vi "PCO Edge_Settings.vi"(10 "Buffers":i16[](array[numeric]), 11 "Handle":u64) -> (3 "Handle Out":u64)   [LabVIEW 2015]
panel:
  in  "Pixel correction":bool
  in  "OK Button":bool
  in  "Pixel clock":u32(ring)=286000000 items=["286MHz"=286000000, "95MHz"=95000000]
  in  "Shutter":u32(ring)=1 items=["Global"=2, "Rolling"=1]
  in  "Binning":u16[](array[numeric])
  in  "ROI":u16[][](array[numeric])
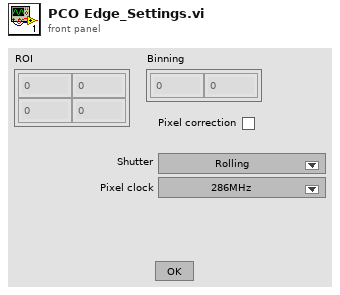
[diagram p1: front panel]
types:
  T1 = cluster{"SSize":u16, "CamType":u16, "CamsSubType":u16, "SerialNumber":u32, "HWVersion":u32, "FWVersion ":u32, "InterfaceType":u16, "HardwareVersions":cluster{"Board":u16, cluster{"string":string, "BatchNumber":u16, "MinorRevision":u8, "MajorRevision":u8, "Variant":u16}[]}, "FirmwareVersions":cluster{"DeviceNum":u16, cluster{"string":string, "MinorRevision":u8, "MajorRevision":u8, "Variant":u16}[]}}
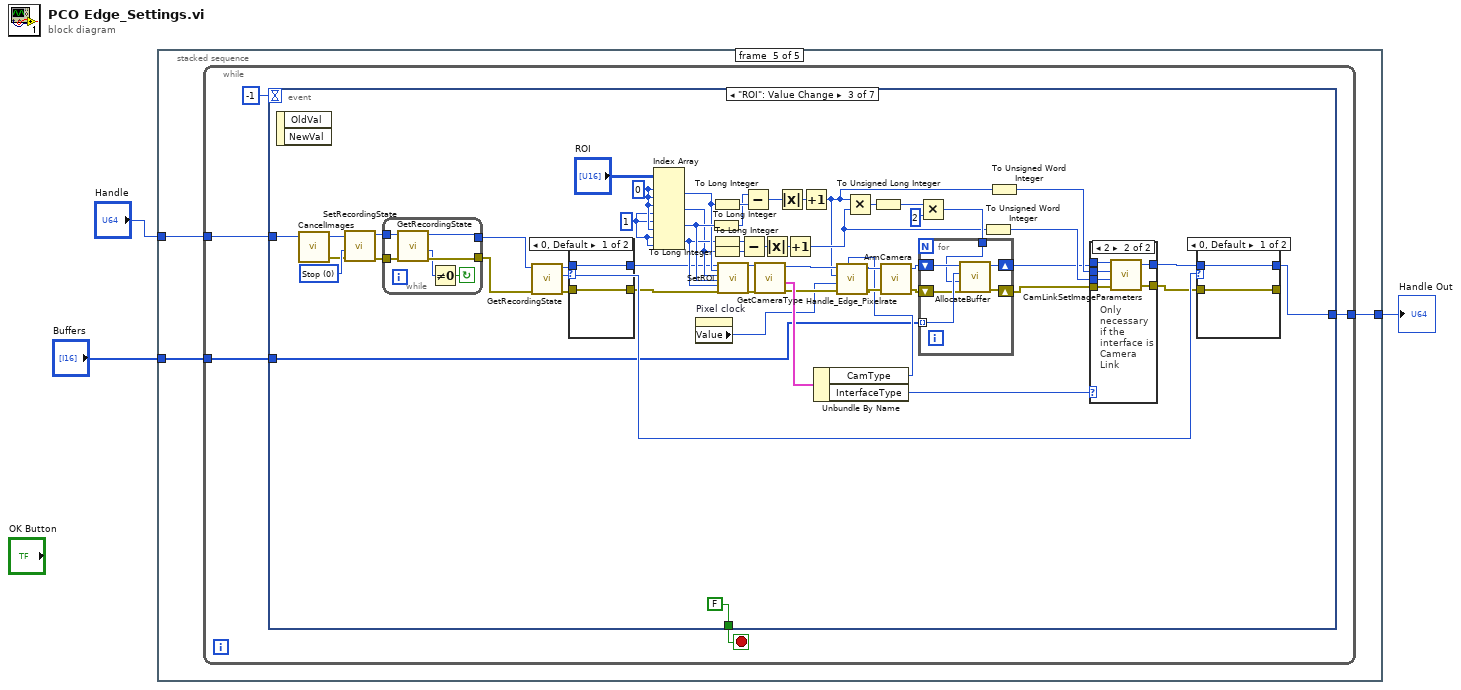
[diagram p0: block diagram]
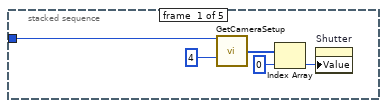
[diagram p2: hidden frame]
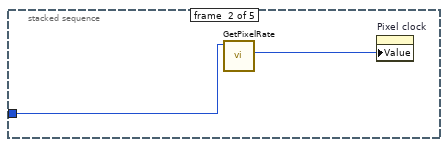
[diagram p3: hidden frame]
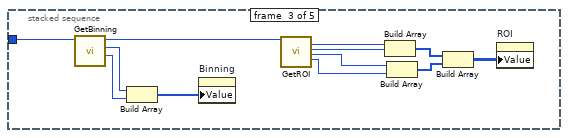
[diagram p4: hidden frame]
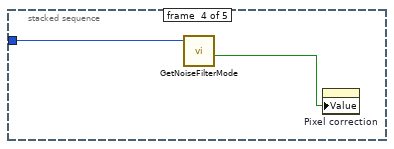
[diagram p5: hidden frame]
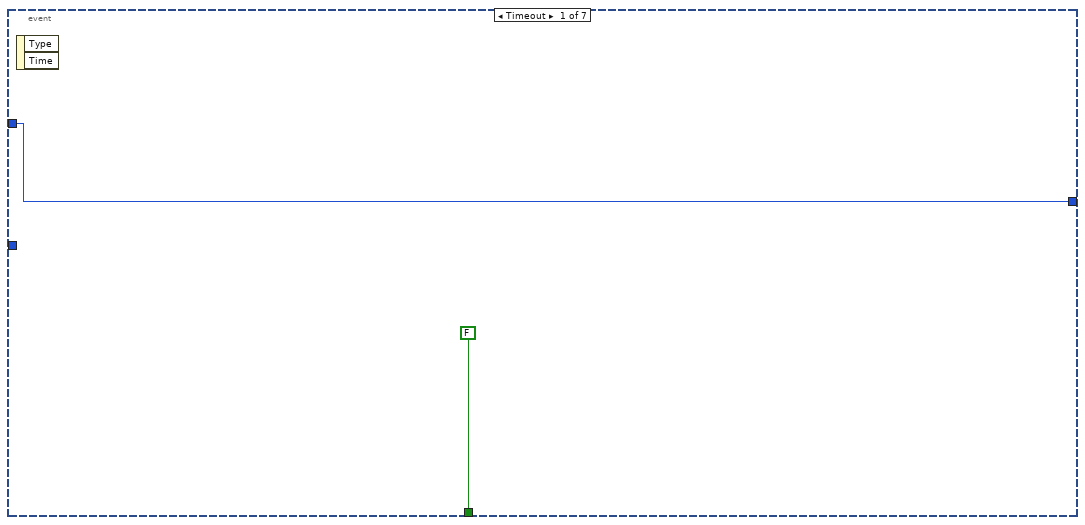
[diagram p6: hidden frame]
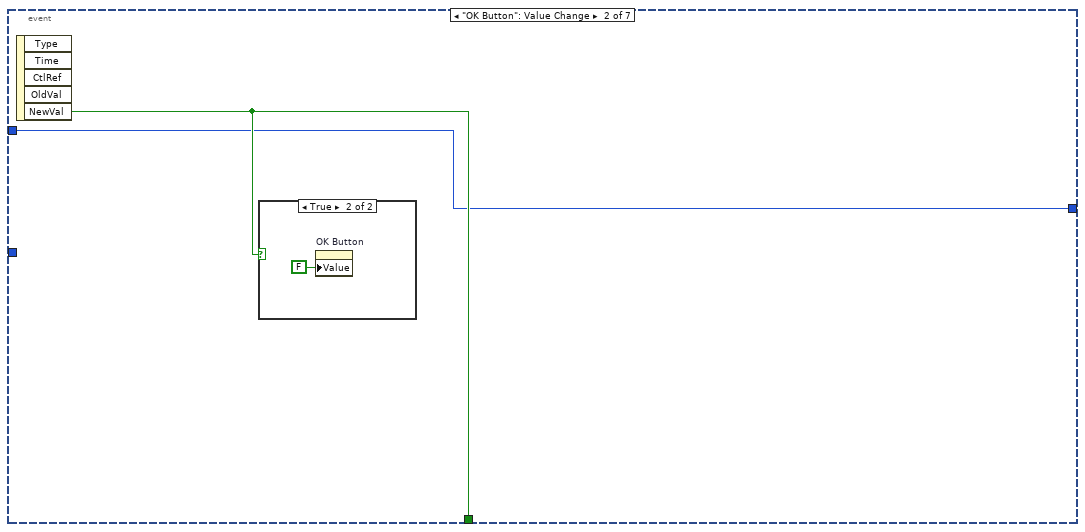
[diagram p7: hidden frame]
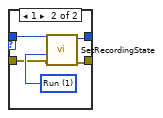
[diagram p10: hidden frame]
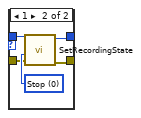
[diagram p11: hidden frame]
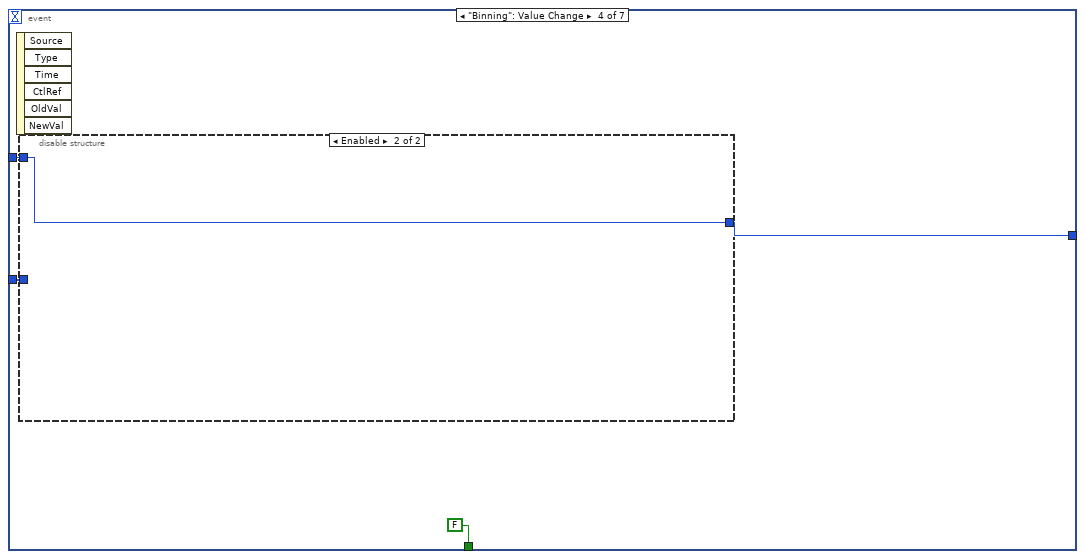
[diagram p12: hidden frame]
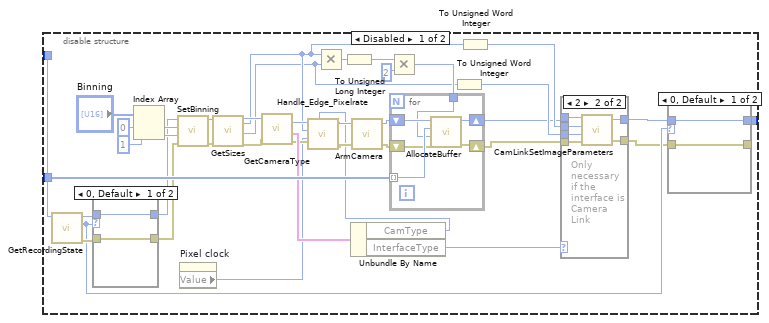
[diagram p13: hidden frame]
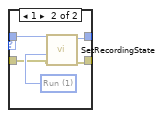
[diagram p15: hidden frame]
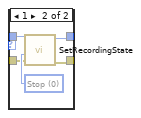
[diagram p16: hidden frame]
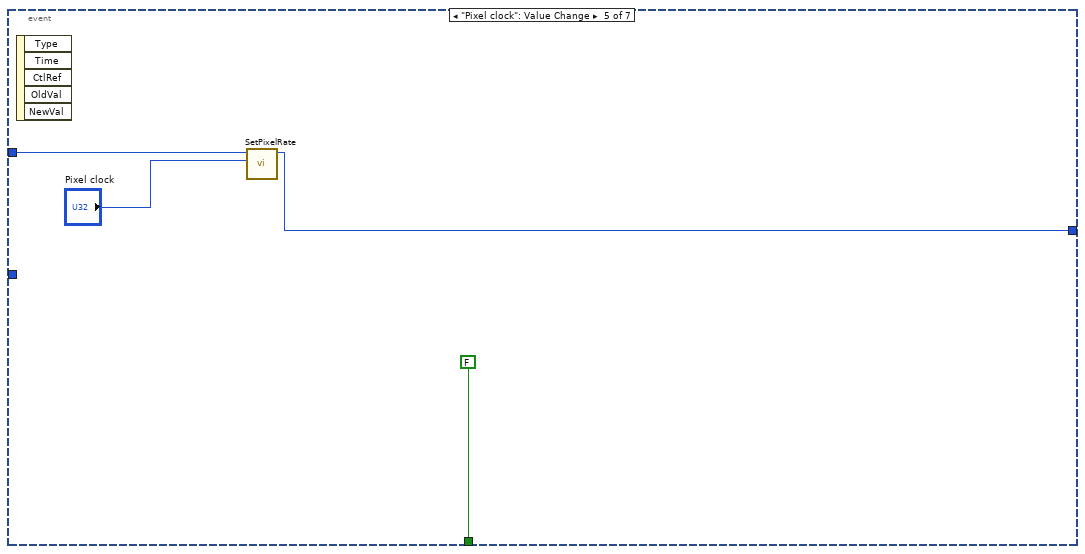
[diagram p17: hidden frame]
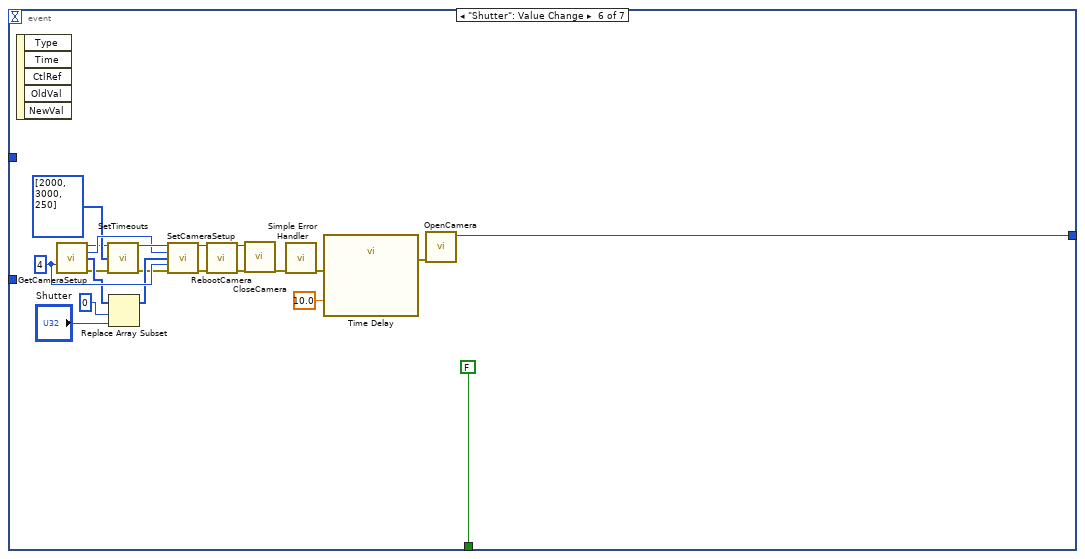
[diagram p18: hidden frame]
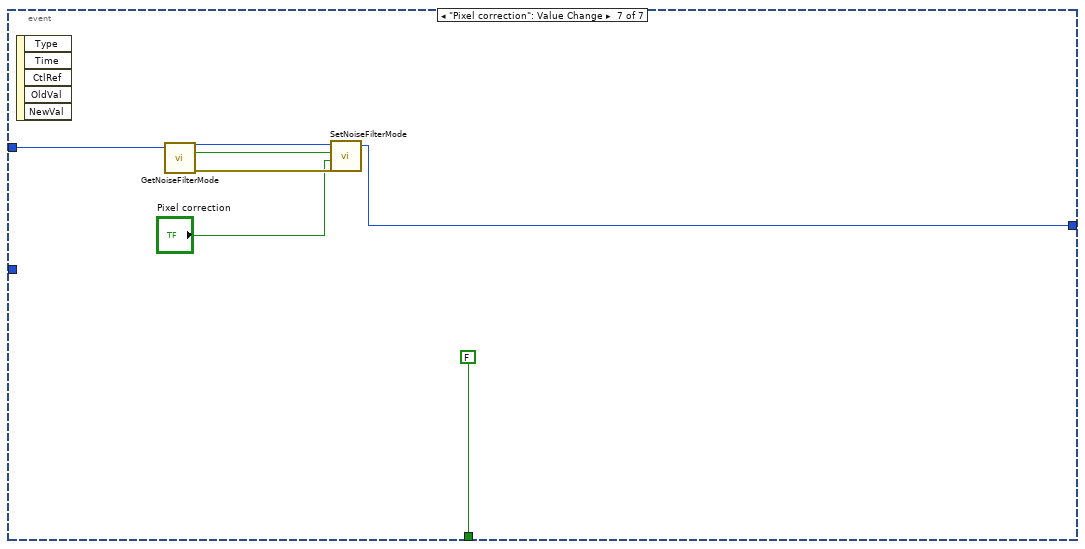
[diagram p19: hidden frame]
diagram:
  n1 = stacked-sequence {
    tunnel: "Handle" -> [w4 w9 w22 w24 w27]
    tunnel: [_ _ _ _ w26] -> w2
    tunnel: "Buffers" -> [_ _ _ _ w25]
    frame #0 {
      n2 = call <userlib>:"GetCameraSetup.vi"("ph"=w4, "Len"=u16 4) -> ("Setup"=w7:u32[])  [unwired: 9 in, 4 out]
      n3 = Index Array(array=w7, index=0) -> (element=w5:u32)
      n4 = property on="Shutter" class="Ring (strict)"("Value"=w5) -> ()  [unwired: 2 in, 2 out]
    }
    frame #1 {
      n5 = call <userlib>:"GetPixelRate.vi"("ph"=w9) -> ("PixelRate"=w10:u32)  [unwired: 3 in, 3 out]
      n6 = property on="Pixel clock" class="Ring (strict)"("Value"=w10) -> ()  [unwired: 2 in, 2 out]
    }
    frame #2 {
      n7 = call <userlib>:"GetBinning.vi"("ph"=w22) -> ("BinVert"=w19:u16, "BinHorz"=w20:u16, "hout"=w21:u64)  [unwired: 4 in, 2 out]
      n8 = Build Array(w20, w19) -> (w18:u16[])
      n9 = property on="Binning" class="Arr (strict)"("Value"=w18) -> ()  [unwired: 2 in, 2 out]
      n10 = call <userlib>:"GetROI.vi"("ph"=w21) -> ("ROIX0"=w16:u16, "ROIY0"=w15:u16, "ROIX1"=w14:u16, "ROIY1"=w13:u16)  [unwired: 13 in, 2 out]
      n11 = Build Array(w16, w15) -> (w12:u16[])
      n12 = Build Array(w14, w13) -> (w17:u16[])
      n13 = Build Array(w12, w17) -> (w11:u16[][])
      n14 = property on="ROI" class="Arr (strict)"("Value"=w11) -> ()  [unwired: 2 in, 2 out]
    }
    frame #3 {
      n15 = call <userlib>:"GetNoiseFilterMode.vi"("ph"=w24) -> ("Hot Pixel Corr"=w23:bool)  [unwired: 2 in, 4 out]
      n16 = property on="Pixel correction" class="Bool (strict)"("Value"=w23) -> ()  [unwired: 2 in, 2 out]
    }
    frame #4 {
      n17 = while {
        tunnel: w27 -> [w30]
        tunnel: [w29] -> w26
        tunnel: w25 -> [w28]
        stop <- w31 stop-if-true
        n18 = event shown="[2] \"ROI\": Value Change" {
          selector: _ -> [_ _ _ _ _ _ _]
          dyn-events: _ -> [_ _ _ _ _ _ _]
          timeout: -1 -> [_ _ _ _ _ _ _]
          tunnel: [FALSE ("NewVal") w36 FALSE ("NewVal") FALSE ("NewVal") FALSE ("NewVal") FALSE ("NewVal") FALSE ("NewVal")] -> w31
          tunnel: w30 -> [w33 w35 w40 w128 w201 _ w227]
          tunnel: [w33 w35 w68 w127 w199 w203 w224] -> w29
          tunnel: w28 -> [_ _ w46 w129 _ _ _]
          event Timeout {
            n19 = event-data() -> ()  [unwired: 1 in, 2 out]
          }
          event "OK Button": Value Change {
            n20 = event-data() -> ("NewVal"=w36:bool)  [unwired: 1 in, 4 out]
            n21 = case shown="True" w36 {
              frame False {
              }
              frame True {
                n22 = property on="OK Button" class="Bool (strict)"("Value"=FALSE ("OK Button")) -> ()  [unwired: 2 in, 2 out]
              }
            }
          }
          event "ROI": Value Change {
            w45 = u16 0 items=["Stop", "Run"] ("RecordingState")
            w89 = 1 ("index (row)")
            w90 = 0 ("index (row)")
            n23 = event-data() -> ()  [unwired: 1 in, 2 out]
            n24 = call <userlib>:"CancelImages.vi"("ph"=w40) -> ("error out"=w42:errorcluster, "hout"=w41:u64)  [unwired: 2 in, 1 out]
            n25 = call <userlib>:"SetRecordingState.vi"("ErrorIn"=w42, "RecordingState"=w45, "ph"=w41) -> ("ErrorOut"=w43:errorcluster, "hout"=w44:u64)  [unwired: 2 in, 1 out]
            n26 = while {
              tunnel: [w96] -> w38
              tunnel: w43 -> [w97]
              tunnel: w44 -> [w98]
              tunnel: [w93] -> w39
              stop <- w94 continue-if-true
              n27 = call <userlib>:"GetRecordingState.vi"("ErrorIn"=w97, "ph"=w98) -> ("ErrorOut"=w96:errorcluster, "RecordingState"=w95:u16, "hout"=w93:u64)  [unwired: 2 in, 1 out]
              n28 = Not Equal To 0?(x=w95) -> (x != 0?=w94:bool)
            }
            n29 = call <userlib>:"GetRecordingState.vi"("ErrorIn"=w38, "ph"=w39) -> ("ErrorOut"=w71:errorcluster, "Error"=w70:i32, "hout"=w72:u64)  [unwired: 2 in, 1 out]
            n30 = case shown="0, Default" w70 {
              tunnel: w72 -> [w115 w119]
              tunnel: w71 -> [w114 w118]
              tunnel: [w115 w117] -> w69
              tunnel: [w114 w116] -> w48
              frame 0, Default {
              }
              frame 1 {
                w120 = u16 0 items=["Stop", "Run"] ("RecordingState")
                n31 = call <userlib>:"SetRecordingState.vi"("ErrorIn"=w118, "RecordingState"=w120, "ph"=w119) -> ("ErrorOut"=w116:errorcluster, "hout"=w117:u64)  [unwired: 2 in, 1 out]
              }
            }
            n32 = Index Array(array="ROI", index (row) #1=w90, index (col) #1=w90, index (row) #2=w90, index (col) #2=w89, index (row) #3=w89, index (col) #3=w90, index (row) #4=w89, index (col) #4=w89) -> (element #1=w84:u16, element #2=w74:u16, element #3=w85:u16, element #4=w75:u16)
            n33 = property on="Pixel clock" class="Ring (strict)"() -> ("Value"=w47:u32)  [unwired: 2 in, 2 out]
            n34 = To Long Integer(number=w85) -> (32bit integer=w81:i32)
            n35 = To Long Integer(number=w84) -> (32bit integer=w82:i32)
            n36 = To Long Integer(number=w75) -> (32bit integer=w77:i32)
            n37 = To Long Integer(number=w74) -> (32bit integer=w76:i32)
            n38 = call <userlib>:"SetROI.vi"("ph"=w69, "ROIX0"=w84, "ROIY0"=w74, "ROIX1"=w85, "ROIY1"=w75, "error in (no error)"=w48) -> ("hout"=w62:u64, "error out"=w61:errorcluster)  [unwired: 12 in]
            n39 = Subtract(x=w77, y=w76) -> (x-y=w78:i32)
            n40 = Subtract(x=w81, y=w82) -> (x-y=w83:i32)
            n41 = call <userlib>:"GetCameraType.vi"("ph"=w62, "error in (no error)"=w61) -> ("hout"=w54:u64, "CameraType"=w60:T1, "error out"=w51:errorcluster)  [unwired: 1 in, 1 out]
            n42 = Absolute Value(x=w78) -> (abs(x)=w79:i32)
            n43 = Absolute Value(x=w83) -> (abs(x)=w80:i32)
            n44 = Increment(x=w79) -> (x+1=w66:i32)
            n45 = Increment(x=w80) -> (x+1=w50:i32)
            n46 = Unbundle By Name(w60) -> ("CamType"=w49:u16, "InterfaceType"=w59:u16)
            n47 = call <userlib>:"Handle_Edge_Pixelrate.vi"("Cameratype"=w49, "error in (no error)"=w51, "PixelRate"=w47, "X-Resolution"=w50, "ph"=w54) -> ("error out"=w52:errorcluster, "hout"=w53:u64)  [unwired: 5 in]
            n48 = Multiply(x=w50, y=w66) -> (x*y=w87:i32)
            n49 = To Unsigned Long Integer(number=w87) -> (unsigned 32bit integer=w73:u32)
            n50 = call <userlib>:"ArmCamera.vi"("error in (no error)"=w52, "ph"=w53) -> ("error out"=w57:errorcluster, "hout"=w58:u64)  [unwired: 1 in, 1 out]
            n51 = Multiply(x=w73, y=u32 2) -> (x*y=w86:u32)
            n52 = for {
              tunnel: w46 -> [w125] mode=indexing
              shift-right: [w122] -> w55
              shift-left: w57 -> [w123]
              shift-right: [w124] -> w56
              shift-left: w58 -> [w126]
              tunnel: w86 -> [w121]
              n53 = call <userlib>:"AllocateBuffer.vi"("error in (no error)"=w123, "Size"=w121, "BufNr"=w125, "ph"=w126) -> ("error out"=w122:errorcluster, "hout"=w124:u64)  [unwired: 2 in, 4 out]
            }
            n54 = To Unsigned Word Integer(number=w66) -> (unsigned 16bit integer=w64:u16)
            n55 = To Unsigned Word Integer(number=w50) -> (unsigned 16bit integer=w65:u16)
            n56 = case shown="2" w59 {
              tunnel: w55 -> [w99 w106]
              tunnel: [w99 w105] -> w63
              tunnel: w56 -> [w100 w104]
              tunnel: [w100 w103] -> w67
              tunnel: w64 -> [_ w102]
              tunnel: w65 -> [_ w101]
              frame 0, Default {
              }
              frame 2 {
                # "Only necessary if the interface is Camera Link"
                n57 = call <userlib>:"CamLinkSetImageParameters.vi"("error in (no error)"=w106, "YRes"=w102, "XRes"=w101, "ph"=w104) -> ("error out"=w105:errorcluster, "hout"=w103:u64)  [unwired: 1 out]
              }
            }
            n58 = case shown="0, Default" w70 {
              tunnel: w67 -> [w108 w112]
              tunnel: w63 -> [w107 w111]
              tunnel: [w108 w110] -> w68
              tunnel: [w107 w109] -> _
              frame 0, Default {
              }
              frame 1 {
                w113 = u16 1 items=["Stop", "Run"] ("RecordingState")
                n59 = call <userlib>:"SetRecordingState.vi"("ErrorIn"=w111, "RecordingState"=w113, "ph"=w112) -> ("ErrorOut"=w109:errorcluster, "hout"=w110:u64)  [unwired: 2 in, 1 out]
              }
            }
          }
          event "Binning": Value Change {
            n60 = event-data() -> ()  [unwired: 1 in, 6 out]
            n61 = disable-structure shown="Enabled" {
              disable-tunnel: w129 -> [w169 _]
              disable-tunnel: w128 -> [w161 w198]
              disable-tunnel: [w160 w198] -> w127
              frame Disabled {
                n62 = call <userlib>:"GetRecordingState.vi"("ph"=w161) -> ("ErrorOut"=w163:errorcluster, "Error"=w162:i32, "hout"=w164:u64)  [unwired: 3 in, 1 out]
                n63 = case shown="0, Default" w162 {
                  tunnel: w164 -> [w186 w190]
                  tunnel: w163 -> [w185 w189]
                  tunnel: [w186 w188] -> w138
                  tunnel: [w185 w187] -> w137
                  frame 0, Default {
                  }
                  frame 1 {
                    w191 = u16 0 items=["Stop", "Run"] ("RecordingState")
                    n64 = call <userlib>:"SetRecordingState.vi"("ErrorIn"=w189, "RecordingState"=w191, "ph"=w190) -> ("ErrorOut"=w187:errorcluster, "hout"=w188:u64)  [unwired: 2 in, 1 out]
                  }
                }
                n65 = Index Array(array="Binning", index #1=0 ("index"), index #2=1 ("index")) -> (element #1=w140:u16, element #2=w139:u16)
                n66 = call "SetBinning.vi"("error in (no error)"=w137, "BinVert"=w139, "BinHorz"=w140, "ph"=w138) -> ("error out"=w133:errorcluster, "hout"=w136:u64)  [unwired: 3 in, 1 out]
                n67 = property on="Pixel clock" class="Ring (strict)"() -> ("Value"=w144:u32)  [unwired: 2 in, 2 out]
                n68 = call <userlib>:"GetSizes.vi"("ph"=w136, "ErrorIn"=w133) -> ("hout"=w135:u64, "XResAct"=w132:u16, "YResAct"=w131:u16, "ErrorOut"=w134:errorcluster)  [unwired: 11 in, 3 out]
                n69 = call <userlib>:"GetCameraType.vi"("ph"=w135, "error in (no error)"=w134) -> ("hout"=w149:u64, "CameraType"=w155:T1, "error out"=w146:errorcluster)  [unwired: 1 in, 1 out]
                n70 = Multiply(x=w132, y=w131) -> (x*y=w167:u16)
                n71 = To Unsigned Long Integer(number=w167) -> (unsigned 32bit integer=w165:u32)
                n72 = Unbundle By Name(w155) -> ("CamType"=w145:u16, "InterfaceType"=w154:u16)
                n73 = call <userlib>:"Handle_Edge_Pixelrate.vi"("Cameratype"=w145, "error in (no error)"=w146, "PixelRate"=w144, "X-Resolution"=w132, "ph"=w149) -> ("error out"=w147:errorcluster, "hout"=w148:u64)  [unwired: 5 in]
                n74 = call <userlib>:"ArmCamera.vi"("error in (no error)"=w147, "ph"=w148) -> ("error out"=w152:errorcluster, "hout"=w153:u64)  [unwired: 1 in, 1 out]
                n75 = Multiply(x=w165, y=u32 2) -> (x*y=w166:u32)
                n76 = for {
                  tunnel: w169 -> [w196] mode=indexing
                  shift-right: [w193] -> w150
                  shift-left: w152 -> [w194]
                  shift-right: [w195] -> w151
                  shift-left: w153 -> [w197]
                  tunnel: w166 -> [w192]
                  n77 = call <userlib>:"AllocateBuffer.vi"("error in (no error)"=w194, "Size"=w192, "BufNr"=w196, "ph"=w197) -> ("error out"=w193:errorcluster, "hout"=w195:u64)  [unwired: 2 in, 4 out]
                }
                n78 = To Unsigned Word Integer(number=w131) -> (unsigned 16bit integer=w157:u16)
                n79 = To Unsigned Word Integer(number=w132) -> (unsigned 16bit integer=w158:u16)
                n80 = case shown="2" w154 {
                  tunnel: w150 -> [w170 w177]
                  tunnel: [w170 w176] -> w156
                  tunnel: w151 -> [w171 w175]
                  tunnel: [w171 w174] -> w159
                  tunnel: w157 -> [_ w173]
                  tunnel: w158 -> [_ w172]
                  frame 0, Default {
                  }
                  frame 2 {
                    # "Only necessary if the interface is Camera Link"
                    n81 = call <userlib>:"CamLinkSetImageParameters.vi"("error in (no error)"=w177, "YRes"=w173, "XRes"=w172, "ph"=w175) -> ("error out"=w176:errorcluster, "hout"=w174:u64)  [unwired: 1 out]
                  }
                }
                n82 = case shown="0, Default" w162 {
                  tunnel: w159 -> [w179 w183]
                  tunnel: w156 -> [w178 w182]
                  tunnel: [w179 w181] -> w160
                  tunnel: [w178 w180] -> _
                  frame 0, Default {
                  }
                  frame 1 {
                    w184 = u16 1 items=["Stop", "Run"] ("RecordingState")
                    n83 = call <userlib>:"SetRecordingState.vi"("ErrorIn"=w182, "RecordingState"=w184, "ph"=w183) -> ("ErrorOut"=w180:errorcluster, "hout"=w181:u64)  [unwired: 2 in, 1 out]
                  }
                }
              }
              frame Enabled {
              }
            }
          }
          event "Pixel clock": Value Change {
            n84 = event-data() -> ()  [unwired: 1 in, 5 out]
            n85 = call <userlib>:"SetPixelRate.vi"("PixelRate"="Pixel clock", "ph"=w201) -> ("hout"=w199:u64)  [unwired: 3 in, 2 out]
          }
          event "Shutter": Value Change {
            w222 = u16 4 ("Len")
            n86 = event-data() -> ()  [unwired: 1 in, 5 out]
            n87 = call <userlib>:"GetCameraSetup.vi"("Len"=w222) -> ("hout"=w206:u64, "Type"=w209:u16, "Setup"=w215:u32[], "error out"=w207:errorcluster)  [unwired: 10 in, 1 out]
            n88 = call <userlib>:"SetTimeouts.vi"("ph"=w206, "Timeouts (ms)"=u32[] [2000, 3000, 250], "error in (no error)"=w207) -> ("hout"=w213:u64, "error out"=w214:errorcluster)  [unwired: 10 in, 1 out]
            n89 = Replace Array Subset(array=w215, new element="Shutter", index=0) -> (w217:u32[])
            n90 = call <userlib>:"SetCameraSetup.vi"("ph"=w213, "Type"=w209, "Setup"=w217, "Len"=w222, "error in (no error)"=w214) -> ("hout"=w210:u64, "error out"=w211:errorcluster)  [unwired: 8 in, 1 out]
            n91 = call <userlib>:"RebootCamera.vi"("ph"=w210, "error in (no error)"=w211) -> ("hout"=w204:u64, "error out"=w205:errorcluster)  [unwired: 11 in, 1 out]
            n92 = call <userlib>:"CloseCamera.vi"("ErrorIn"=w205, "Handle in"=w204) -> ("ErrorOut"=w212:errorcluster)  [unwired: 1 in, 2 out]
            n93 = call <vilib>:"Simple Error Handler.vi"("error in (no error)"=w212) -> ("error out"=w218:errorcluster)  [unwired: 4 in, 4 out]
            n94 = call "Time Delay"("error in (no error)"=w218, "Delay Time (s)"=10.0) -> ("error out"=w220:errorcluster)  [unwired: 9 in]
            n95 = call <userlib>:"OpenCamera.vi"("ErrorIn"=w220) -> ("Handle out"=w203:u64)  [unwired: 3 in, 3 out]
          }
          event "Pixel correction": Value Change {
            n96 = event-data() -> ()  [unwired: 1 in, 5 out]
            n97 = call <userlib>:"GetNoiseFilterMode.vi"("ph"=w227) -> ("hout"=w228:u64, "Noise Filter"=w225:bool, "error out"=w229:errorcluster)  [unwired: 2 in, 2 out]
            n98 = call <userlib>:"SetNoiseFilterMode.vi"("error in (no error)"=w229, "Hot Pixel Corr"="Pixel correction", "Noise Filter"=w225, "ph"=w228) -> ("hout"=w224:u64)  [unwired: 2 out]
          }
        }
      }
    }
  }
  "Handle Out" <- w2
